vi "MonoSpec50 MessageBox.vi"(4 "error in (no error)":errorcluster, 7 "End":refnum<vi>) -> (0 "error out":errorcluster)   [LabVIEW 2012]
panel:
  # "Veuillez patientez pendant que le monochromateur recherche une position de référence.\nCela peut prendre jusqu'à 25s..."
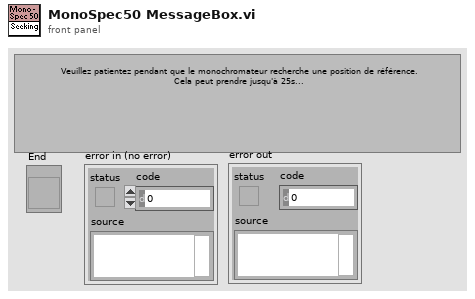
[diagram p1: front panel]
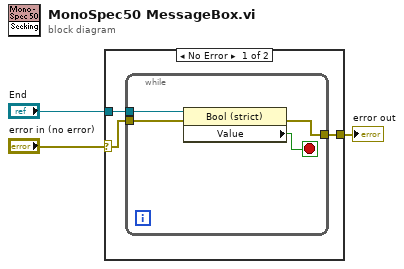
[diagram p0: block diagram]
diagram:
  n1 = case shown="No Error" "error in (no error)" {
    selector: "error in (no error)" -> [w4 w11]
    tunnel: [w6 w11] -> w3
    tunnel: "End" -> [w5 _]
    frame No Error {
      n2 = while {
        tunnel: [w8] -> w6
        tunnel: w5 -> [w9]
        tunnel: w4 -> [w7]
        stop <- w10 stop-if-true
        n3 = property class="Bool (strict)"(reference=w9, error in=w7) -> (error out=w8:errorcluster, "Value"=w10:bool)  [unwired: 1 out]
      }
    }
    frame Error {
    }
  }
  "error out" <- w3
